vi "Remove GObject.vi"(8 "error in (no error)":errorcluster, 10 "GObject UID":string, 11 "VI Data in":refnum<class "VI Data.lvclass">) -> (0 "error out":errorcluster, 1 "Removed GObject":refnum<class "GObject.lvclass">, 2 "found":bool, 3 "VI Data out":refnum<class "VI Data.lvclass">)   [LabVIEW 2013, in "SET Project Data.lvlib" / "VI Data.lvclass"]
uses:
  VI Data.lvclass
  Control Classes/GObject/GObject.lvclass
  VI Data.lvclass/VI Data.ctl
  Control Classes/GObject/Read UID.vi
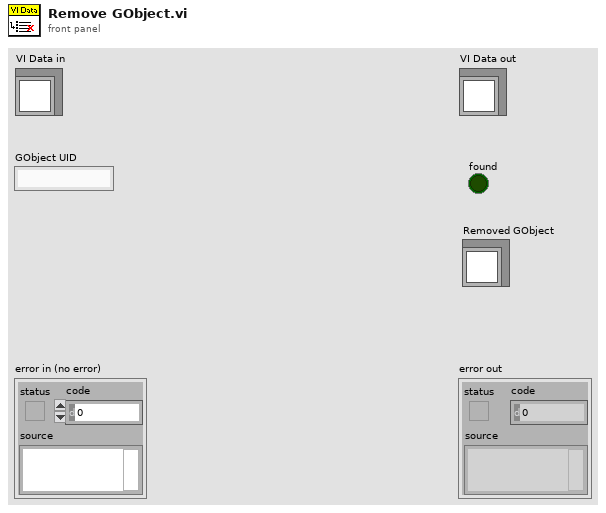
[diagram p1: front panel]
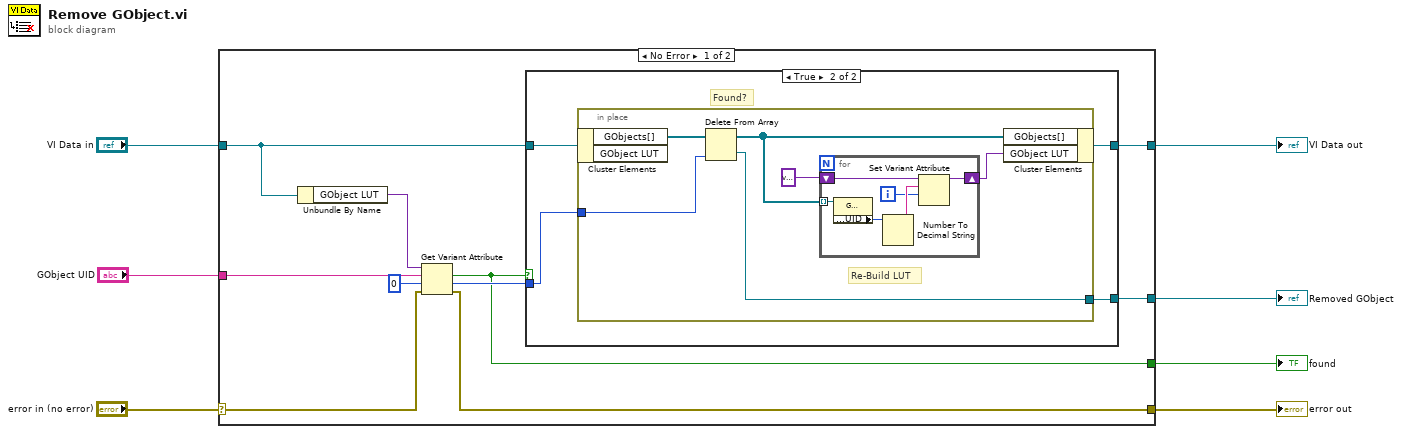
[diagram p0: block diagram]
diagram:
  n1 = case shown="No Error" "error in (no error)" {
    selector: "error in (no error)" -> [w12 w36]
    tunnel: [w11 w36] -> w6
    tunnel: [w10 w35] -> w4
    tunnel: "VI Data in" -> [w14 w35]
    tunnel: "GObject UID" -> [w15 _]
    tunnel: [w9 _] -> w2
    tunnel: [w8 _] -> w1
    frame No Error {
      n2 = Unbundle By Name(w14) -> ("GObject LUT"=w16:variant)
      n3 = Get Variant Attribute(Variant=w16, name=w15, default value (empty Variant)=0, error in=w12) -> (found=w9:bool, value=w13:i32, error out=w11:errorcluster)  [unwired: 1 out]
      n4 = case shown="True" w9 {
        tunnel: w14 -> [w18 w22]
        tunnel: w13 -> [_ w21]
        tunnel: [_ w20] -> w8
        tunnel: [w18 w19] -> w10
        frame False {
        }
        frame True {
          # "Found?"
          n5 = in-place {
            in-place-border: w21 -> [w27]
            in-place-border: [w26] -> w20
            # "Re-Build LUT"
            n6 = in-place-cluster #1(w22) -> ("GObjects[]"=w28:refnum<class "GObject.lvclass">[])  [unwired: 1 out]
            n7 = Delete From Array(array=w28, index=w27) -> (deleted portion=w26:refnum<class "GObject.lvclass">, array with subset deleted=w25:refnum<class "GObject.lvclass">[])  [unwired: 1 in]
            n8 = for {
              tunnel: w25 -> [w32] mode=indexing
              shift-right: [w33] -> w23
              shift-left: variant ("type") -> [w34]
              i -> [w29]
              n9 = property class="GObject.lvclass"(reference=w32) -> ("Properties:UID"=w31:i32)  [unwired: 1 in, 2 out]
              n10 = Number To Decimal String(number=w31) -> (decimal integer string=w30:string)  [unwired: 1 in]
              n11 = Set Variant Attribute(Variant=w34, name=w30, value=w29) -> (Variant out=w33:variant)  [unwired: 1 in, 2 out]
            }
            n12 = in-place-cluster #1("GObjects[]"=w25, "GObject LUT"=w23) -> (w19:refnum<class "VI Data.lvclass">)
          }
        }
      }
    }
    frame Error {
    }
  }
  "error out" <- w6
  "VI Data out" <- w4
  "found" <- w2
  "Removed GObject" <- w1
